vi "GooglePlatform OAuth Test.vi"() -> ()   [LabVIEW 2013]
uses:
  Oauth2/Oauth2.lvclass/Oauth2.ctl
  Oauth2.Google/Oauth2.Google.lvclass
  Oauth2/Read RefreshToken.vi
  Oauth2/Read ExpiresIn.vi
  Oauth2/Read Redirect URI.vi
  Oauth2/Read scopes.vi
  <vilib>/dlg_ctls.llb/Space Constant.vi
  OAuthToken/Retrieve Element.vi
  Oauth2/Oauth2.lvclass
  <vilib>/LabVIEW Open Source Project/OpenURI/uri/URI.lvclass
  <vilib>/httpClient/LabVIEWHTTPClient.lvlib
panel:
  in  "relative API URI":string="userinfo/v2/me"
  out "REST API Error":errorcluster
  in  "Query API Version":bool
  in  "Refresh":bool
  in  "Authorize":bool
  out "API Response":string
  out "HTTP Response Headers":string
  out "Redirect URI":string
  out "scopes":string[](array[string])
  out "Expires In":u32
  out "Refresh Token":string
  in  "Google Client Secret":string
  in  "Google Client ID":string
  out "Google Access Token":string
  out "Oauth Error":errorcluster
  # "Google Cloud Application API Access Example"
  # "G Open Source Project for LabVIEW\nhttps://github.com/LabVIEW-Open-Source/Oauth2"
  # "1- Get a Client ID and Client Secret from the application's admin. \n\n          * To access your own server, log into your site, create an application and set the access scope.\n             you want. \n          * This Oauth2.0 API uses the following redirect URL: http://localhost:58888/Oauth2/Redirect\n          * Record the client ID and client secret and fill in the fields below."
  # "2- Get an Access Token. You will be redirected your Google's Authorization Server URI\n              * Use the \"Get Access Token\" button on the top right of this page.\n\n3- Once you have authenticated yourself, you will receive an access token.\n              * Use the \"Refresh Token\" button to request a fresh token\n                       OR\n              * Use the Access Token to query the Google API (example is to retrieve the User Info)\n\n4- Visit \"https://developers.google.com/oauthplayground/\" if you'd like to run Oauth2 tests."
  # "0: Never expired"
  # "https://www.googleapis.com/"
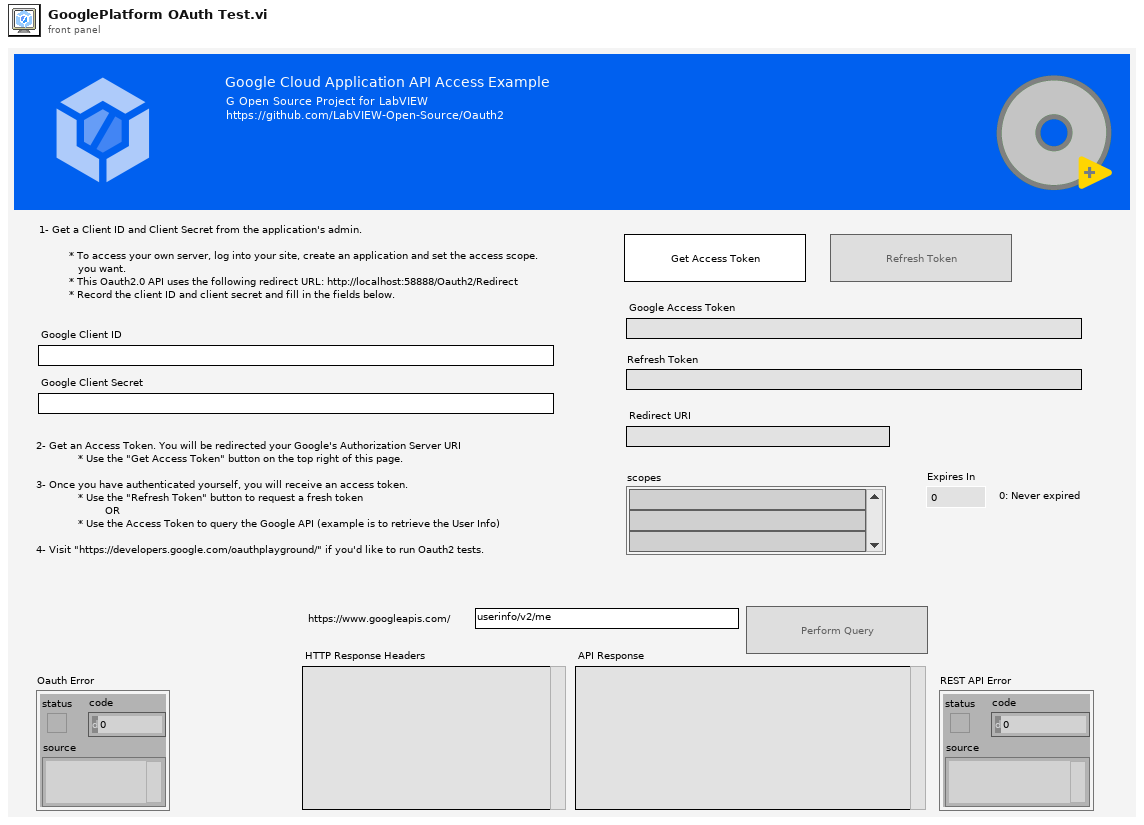
[diagram p1: front panel]
types:
  T1 = enum8{"Enabled", "Disabled", "Disabled and Grayed Out"}
  T2 = typedef "LabVIEWHTTPClient.lvlib/ClientHandle.ctl" = refnum<k1>
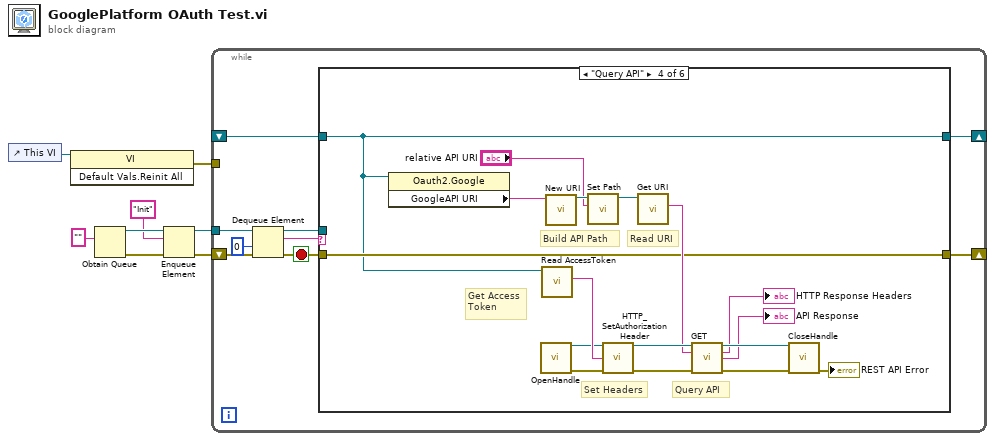
[diagram p0: block diagram]
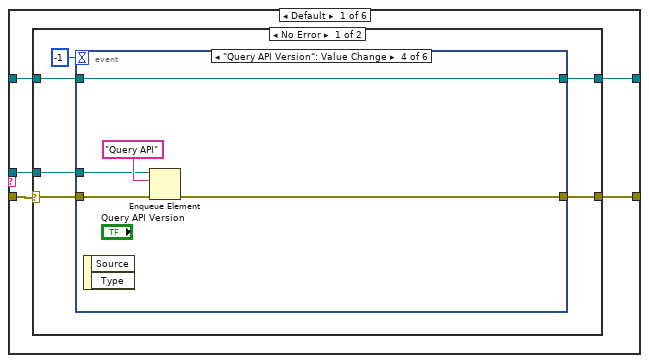
[diagram p2: hidden frame]
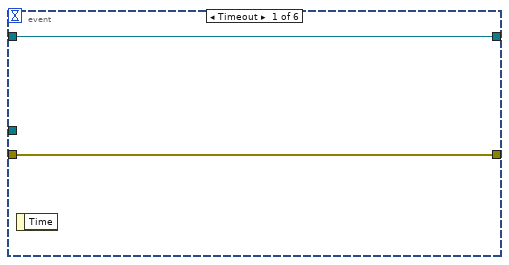
[diagram p3: hidden frame]
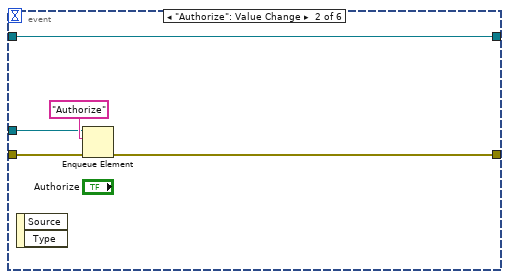
[diagram p4: hidden frame]
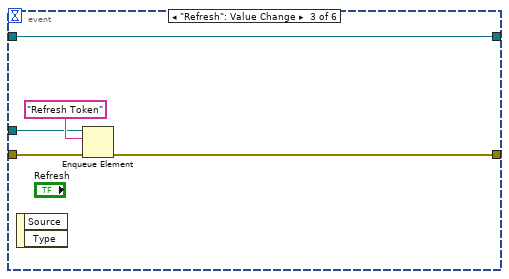
[diagram p5: hidden frame]
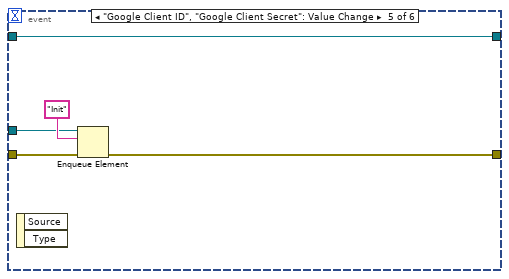
[diagram p6: hidden frame]
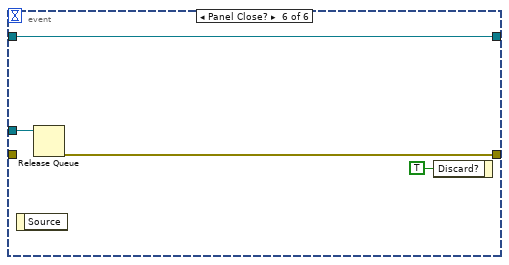
[diagram p7: hidden frame]
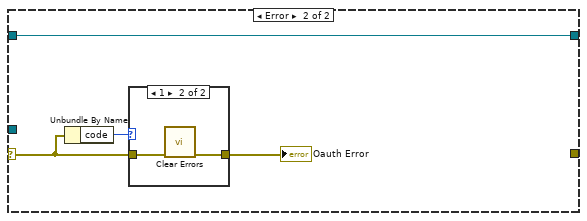
[diagram p8: hidden frame]
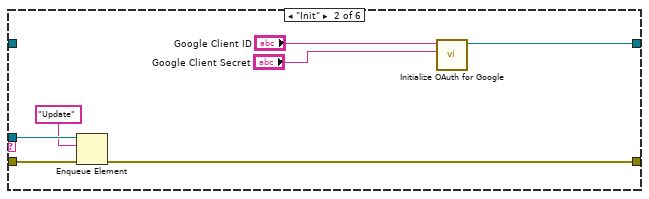
[diagram p10: hidden frame]
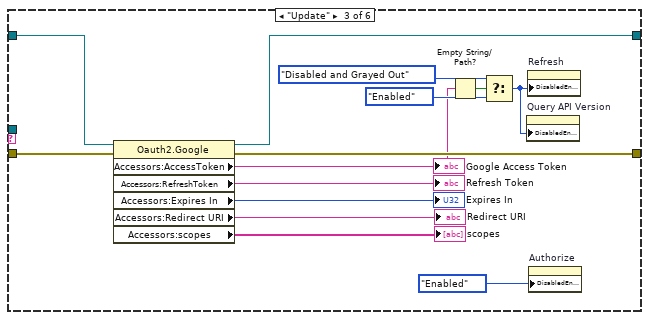
[diagram p11: hidden frame]
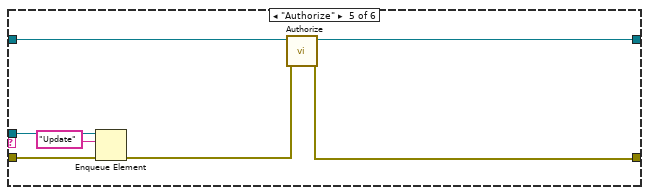
[diagram p12: hidden frame]
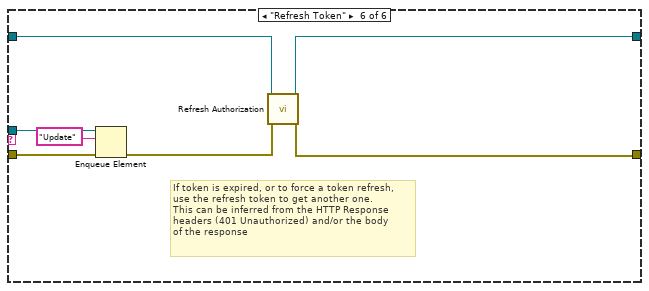
[diagram p13: hidden frame]
diagram:
  n1 = control-ref of="This VI"() -> (w1:refnum<vi>)
  n2 = invoke class="VI" method="Default Vals.Reinit All"(reference=w1) -> (error out=w2:errorcluster)  [unwired: 2 in, 2 out]
  n3 = Obtain Queue(element data type="") -> (queue out=w5:refnum<queue>, error out=w7:errorcluster)  [unwired: 4 in, 1 out]
  n4 = Enqueue Element(queue=w5, element="Init", error in (no error)=w7) -> (queue out=w4:refnum<queue>, error out=w6:errorcluster)  [unwired: 1 in, 1 out]
  n5 = while {
    tunnel: w4 -> [w17]
    shift-right: [w12] -> _
    shift-left: _ -> [w11]
    shift-right: [w9] -> _
    shift-left: w6 -> [w13]
    tunnel: w2 -> [_]
    stop <- w10 stop-if-true
    n6 = Dequeue Element(queue=w17, timeout in ms (-1)=0, error in (no error)=w13) -> (queue out=w14:refnum<queue>, element=w15:string, error out=w10:errorcluster)  [unwired: 1 out]
    n7 = case shown="\"Query API\"" w15 {
      tunnel: w14 -> [w22 w68 _ _ w104 w112]
      tunnel: [w21 w62 w69 w85 w100 w107] -> w12
      tunnel: w11 -> [w20 _ w71 w85 w101 w108]
      tunnel: w10 -> [w19 w65 w79 w88 w103 w111]
      tunnel: [w18 w66 w78 w88 w106 w109] -> w9
      frame Default {
        n8 = case shown="No Error" w19 {
          selector: w19 -> [w23 w57]
          tunnel: w22 -> [w27 _]
          tunnel: [w26 w58] -> w21
          tunnel: w20 -> [w25 w58]
          tunnel: [w24 _] -> w18
          frame No Error {
            n9 = event shown="[3] \"Query API Version\": Value Change" {
              selector: _ -> [_ _ _ _ _ _]
              dyn-events: _ -> [_ _ _ _ _ _]
              timeout: -1 -> [_ _ _ _ _ _]
              tunnel: w27 -> [_ w34 w39 w44 w49 w54]
              tunnel: [w30 w32 w37 w42 w47 w52] -> w26
              tunnel: w25 -> [w30 w32 w37 w42 w47 w52]
              tunnel: [w29 w31 w36 w41 w46 w51] -> w24
              tunnel: w23 -> [w29 w33 w38 w43 w48 _]
              event Timeout {
                n10 = event-data() -> ()  [unwired: 1 in, 1 out]
              }
              event "Authorize": Value Change {
                n11 = event-data() -> ()  [unwired: 1 in, 2 out]
                n12 = Enqueue Element(queue=w34, element="Authorize", error in (no error)=w33) -> (error out=w31:errorcluster)  [unwired: 1 in, 2 out]
              }
              event "Refresh": Value Change {
                n13 = event-data() -> ()  [unwired: 1 in, 2 out]
                n14 = Enqueue Element(queue=w39, element="Refresh Token", error in (no error)=w38) -> (error out=w36:errorcluster)  [unwired: 1 in, 2 out]
              }
              event "Query API Version": Value Change {
                n15 = event-data() -> ()  [unwired: 1 in, 2 out]
                n16 = Enqueue Element(queue=w44, element="Query API", error in (no error)=w43) -> (error out=w41:errorcluster)  [unwired: 1 in, 2 out]
              }
              event "Google Client ID", "Google Client Secret": Value Change {
                n17 = event-data() -> ()  [unwired: 1 in, 2 out]
                n18 = Enqueue Element(queue=w49, element="Init", error in (no error)=w48) -> (error out=w46:errorcluster)  [unwired: 1 in, 2 out]
              }
              event Panel Close? {
                n19 = event-data() -> ()  [unwired: 1 in, 1 out]
                n20 = Release Queue(queue=w54) -> (error out=w51:errorcluster)  [unwired: 2 in, 2 out]
                n21 = event-data("Discard?"=TRUE) -> ()  [unwired: 1 in, 1 out]
              }
            }
          }
          frame Error {
            n22 = Unbundle By Name(w57) -> ("code"=w55:i32)
            n23 = case shown="1" w55 {
              tunnel: w57 -> [w59 w61]
              tunnel: [w59 w60] -> w56
              frame Default {
              }
              frame 1 {
                n24 = call <vilib>:"Clear Errors.vi"("error in (no error)"=w61) -> ("error out"=w60:errorcluster)  [unwired: 6 in]
              }
            }
            "Oauth Error" <- w56
          }
        }
      }
      frame "Init" {
        n25 = Enqueue Element(queue=w68, element="Update", error in (no error)=w65) -> (error out=w66:errorcluster)  [unwired: 1 in, 2 out]
        n26 = call "Initialize OAuth for Google.vi"("Client Secret"="Google Client Secret", "Client ID"="Google Client ID") -> ("Oauth2.Google"=w62:refnum<class "Oauth2.Google.lvclass">)  [unwired: 8 in, 1 out]
      }
      frame "Update" {
        n27 = property class="Oauth2.Google"(reference=w71, error in=w79) -> (reference out=w69:refnum<class "Oauth2.Google.lvclass">, error out=w78:errorcluster, "Accessors:AccessToken"=w77:string, "Accessors:RefreshToken"=→"Refresh Token":string, "Accessors:Expires In"=→"Expires In":u32, "Accessors:Redirect URI"=→"Redirect URI":string, "Accessors:scopes"=→"scopes":string[])
        "Google Access Token" <- w77
        n28 = Empty String/Path?(string/path=w77) -> (empty?=w82:bool)
        n29 = Select(t=T1."Disabled and Grayed Out" ("Disabled"), s=w82, f=T1."Enabled" ("Disabled")) -> (s? t:f=w72:T1)
        n30 = property on="Query API Version" class="Bool"("DisabledEnum"=w72) -> ()  [unwired: 2 in, 2 out]
        n31 = property on="Refresh" class="Bool"("DisabledEnum"=w72) -> ()  [unwired: 2 in, 2 out]
        n32 = property on="Authorize" class="Bool"("DisabledEnum"=T1."Enabled" ("Disabled")) -> ()  [unwired: 2 in, 2 out]
      }
      frame "Query API" {
        # "Query API"
        # "Set Headers"
        # "Get Access\nToken"
        # "Read URI"
        # "Build API Path"
        n33 = property class="Oauth2.Google"(reference=w85) -> ("GoogleAPI URI"=w84:string)  [unwired: 1 in, 2 out]
        n34 = call <vilib>:"OpenHandle.vi"() -> ("client handle out"=w98:T2, "error out"=w93:errorcluster)  [unwired: 14 in]
        n35 = call "Read AccessToken.vi"("Oauth2 in"=w85) -> ("Access Token"=w99:string)  [unwired: 8 in, 2 out]
        n36 = call <vilib>:"New URI.vi"("URI"=w84) -> ("URI"=w96:refnum<class "URI.lvclass">)  [unwired: 9 in, 1 out]
        n37 = call <vilib>:"Set Path.vi"("path"="relative API URI", "URI in"=w96) -> ("URI out"=w97:refnum<class "URI.lvclass">)  [unwired: 8 in, 1 out]
        n38 = call "HTTP_SetAuthorizationHeader.vi"("Client Handle"=w98, "Access Token"=w99, "error in (no error)"=w93) -> ("client handle dup"=w95:T2, "error out"=w92:errorcluster)  [unwired: 11 in]
        n39 = call <vilib>:"Get URI.vi"("URI in"=w97) -> ("URI String"=w94:string)  [unwired: 8 in, 2 out]
        n40 = call <vilib>:"GET.vi"("client handle"=w95, "url"=w94, "error in (no error)"=w92) -> ("client handle out"=w91:T2, "headers"=→"HTTP Response Headers":string, "body"=→"API Response":string, "error out"=w90:errorcluster)  [unwired: 9 in]
        n41 = call <vilib>:"CloseHandle.vi"("client handle"=w91, "error in (no error)"=w90) -> ("error out"=→"REST API Error":errorcluster)  [unwired: 13 in]
      }
      frame "Authorize" {
        n42 = Enqueue Element(queue=w104, element="Update", error in (no error)=w103) -> (error out=w102:errorcluster)  [unwired: 1 in, 2 out]
        n43 = call "Authorize.vi"("error in (no error)"=w102, "Oauth2 in"=w101) -> ("error out"=w106:errorcluster, "Oauth2 out"=w100:refnum<class "Oauth2.Google.lvclass">)  [unwired: 7 in, 1 out]
      }
      frame "Refresh Token" {
        # "If token is expired, or to force a token refresh, \nuse the refresh token to get another one.\nThis can be inferred from the HTTP Response\nheaders (401 Unauthorized) and/or the body\nof the response"
        n44 = Enqueue Element(queue=w112, element="Update", error in (no error)=w111) -> (error out=w110:errorcluster)  [unwired: 1 in, 2 out]
        n45 = call "Refresh Authorization.vi"("error in (no error)"=w110, "Oauth2 in"=w108) -> ("error out"=w109:errorcluster, "Oauth2 out"=w107:refnum<class "Oauth2.Google.lvclass">)  [unwired: 7 in, 1 out]
      }
    }
  }
